vi "Cmd and Reply.vi"(8 "error in (no error)":errorcluster, 9 "EtherCAT command":T3 {"Bank" format="%.0x"; "Type" format="%.0x"; "Cmd" items=["NONE", "ROR", "ROL", "MST", "MVP", "SAP", "GAP", "STAP", "RSAP", "SGP", "GGP"]; "Module" format="%.0x"}, 10 "nodeAddr in":u16 format="%.0x", 11 "masterHdl in":T2) -> (0 "error out":errorcluster, 1 "EtherCAT reply":T1 {"Cmd" format="%.0x"}, 2 "nodeAddr out":u16 format="%.0x", 3 "masterHdl out":T2, 5 "raw data":u8[](array[numeric]))   [LabVIEW 2017, in "NI_Robotics_KUKA youBot Host.lvlib"]
uses:
  <vilib>/robotics/KUKA youBot/NI_Robotics_KUKA youBot Host.lvlib
  <vilib>/robotics/KUKA youBot/EtherCAT/EtherCAT Command.ctl
  <vilib>/robotics/KUKA youBot/EtherCAT/CmdCtrls/Param Cmd.ctl
  <vilib>/robotics/KUKA youBot/EtherCAT/LowLevel/Mater Handler.ctl
  <vilib>/robotics/KUKA youBot/EtherCAT/EtherCAT Reply.ctl
  <vilib>/robotics/Utilities/NI_Robotics Utilities.lvlib
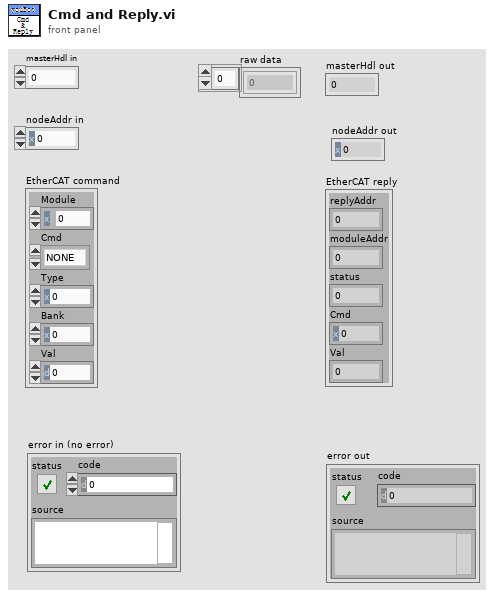
[diagram p1: front panel]
types:
  T1 = typedef "NI_Robotics_KUKA youBot Host.lvlib/EtherCAT Reply.ctl" = cluster{"replyAddr":u8, "moduleAddr":u8, "status":u8, "Cmd":u8, "Val":i32}
  T2 = typedef "NI_Robotics_KUKA youBot Host.lvlib/Mater Handler.ctl" = i32
  T3 = typedef "NI_Robotics_KUKA youBot Host.lvlib/EtherCAT Command.ctl" = cluster{"Module":u8, "Cmd":T4, "Type":u8, "Bank":u8, "Val":u32}
  T4 = typedef "NI_Robotics_KUKA youBot Host.lvlib/Param Cmd.ctl" = u8
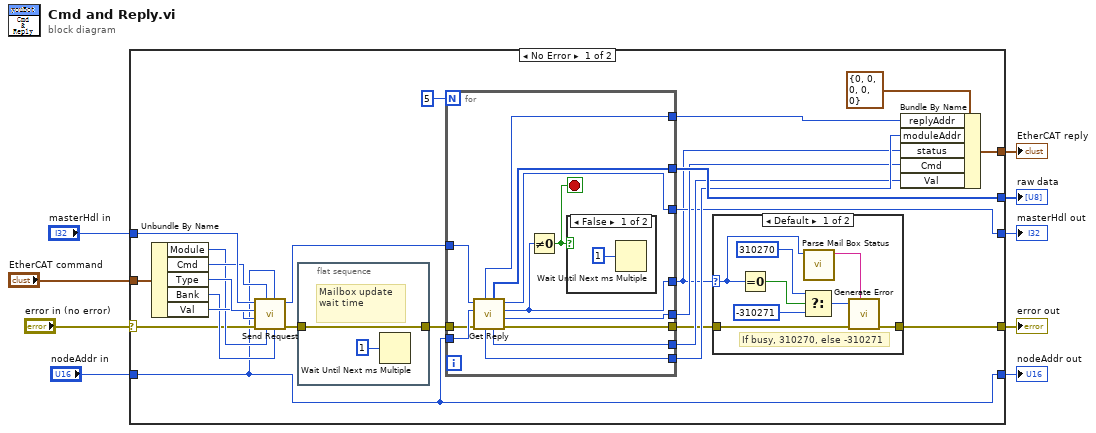
[diagram p0: block diagram]
diagram:
  n1 = case shown="No Error" "error in (no error)" {
    selector: "error in (no error)" -> [w26 w58]
    tunnel: "masterHdl in" -> [w33 w60]
    tunnel: "nodeAddr in" -> [w16 w59]
    tunnel: "EtherCAT command" -> [w32 _]
    tunnel: [w24 _] -> w5
    tunnel: [w10 w58] -> w4
    tunnel: [w18 _] -> w3
    tunnel: [w17 w60] -> w2
    tunnel: [w16 w59] -> w1
    frame No Error {
      n2 = Unbundle By Name(w32) -> ("Module"=w28:u8, "Cmd"=w30:T4, "Type"=w31:u8, "Bank"=w27:u8, "Val"=w29:u32)
      n3 = call <vilib>:"Send Request.vi"("bank"=w27, "nodeAddr"=w16, "module"=w28, "cmd"=w30, "error in (no error)"=w26, "value"=w29, "type"=w31, "masterHdl in"=w33) -> ("error out"=w13:errorcluster, "master ref out"=w25:T2)  [unwired: 2 in]
      n4 = flat-sequence {
        tunnel: [w43] -> w14
        tunnel: w13 -> [w43]
        frame #0 {
          # "Mailbox update wait time"
          n5 = Wait Until Next ms Multiple(millisecond multiple=u32 1) -> ()  [unwired: 1 out]
        }
      }
      n6 = for {
        N: 5 -> [_]
        tunnel: w25 -> [w56]
        tunnel: [w55] -> w24
        tunnel: [w54] -> w22
        tunnel: [w53] -> w21
        tunnel: [w52] -> w20
        tunnel: [w46] -> w12
        tunnel: [w51] -> w19
        tunnel: [w50] -> w17
        tunnel: w16 -> [w49]
        tunnel: w14 -> [w48]
        tunnel: [w47] -> w11
        stop <- w45 stop-if-true
        n7 = call <vilib>:"Get Reply.vi"("error in (no error)"=w48, "node address"=w49, "masterHdl in"=w56) -> ("error out"=w47:errorcluster, "Cmd"=w51:T4, "status"=w46:u8, "master ref out"=w50:T2, "value"=w52:i32, "raw data"=w55:u8[], "module adr"=w53:u8, "reply addr"=w54:u8)  [unwired: 1 in]
        n8 = Not Equal To 0?(x=w46) -> (x != 0?=w45:bool)
        n9 = case shown="False" w45 {
          frame False {
            n10 = Wait Until Next ms Multiple(millisecond multiple=u32 1) -> ()  [unwired: 1 out]
          }
          frame True {
          }
        }
      }
      n11 = case shown="Default" w12 {
        selector: w12 -> [w38 _]
        tunnel: w11 -> [w40 w42]
        tunnel: [w39 w42] -> w10
        frame Default {
          # "If busy, 310270, else -310271"
          n12 = Equal To 0?(x=w38) -> (x = 0?=w37:bool)
          n13 = Select(t=310270, s=w37, f=-310271 ("code")) -> (s? t:f=w34:i32)
          n14 = call <vilib>:"Parse Mail Box Status.vi"("status"=w38) -> ("Status Meaning"=w41:string)  [unwired: 10 in]
          n15 = call <vilib>:"Generate Error.vi"("<append> (\"\")"=w41, "error in (no error)"=w40, "code"=w34) -> ("error out"=w39:errorcluster)  [unwired: 8 in]
        }
        frame 100 {
        }
      }
      n16 = Bundle By Name(cluster=T1 {"replyAddr"=0, "moduleAddr"=0, "status"=0, "Cmd"=0, "Val"=0} ("EtherCAT Reply"), "replyAddr"=w22, "moduleAddr"=w21, "status"=w12, "Cmd"=w19, "Val"=w20) -> (w18:T1)
    }
    frame Error {
    }
  }
  "masterHdl out" <- w2
  "nodeAddr out" <- w1
  "EtherCAT reply" <- w3
  "error out" <- w4
  "raw data" <- w5
